vi "epx_Update Vector Color.vi"(8 "error in (no error)":errorcluster, 9 "Background Decoratin":refnum<vi>, 10 "Display State In":T1={"BGColor"=0, "FGColor"=0, "GridColor"=9868950, "Number of Polar Grids"=12, "Number of Circle Grids"=4, "Vector.Active"=0, "Vectors.Properties"=[], "Height"=0, "Width"=0} {"Number of Circle Grids" min=1 max=100 step=1; "Number of Polar Grids" min=1 max=100 step=1}, 11 "Vector Diagram":refnum<vi>) -> (0 "error out":errorcluster, 1 "Background Decoratin out":refnum<vi>, 3 "Vector Diagram out":refnum<vi>)   [LabVIEW 2011, in "NI_EP_Basic.lvlib" / "EPX Vector Diagram.xctl"]
uses:
  <vilib>/addons/Electrical Power/Basic/Controls/Vector Diagram/EPX Vector Diagram.xctl
  <vilib>/addons/Electrical Power/Basic/Controls/Vector Diagram/Abilities/epx_Vector Diagram State.ctl
  <vilib>/addons/Electrical Power/Basic/Controls/Vector Diagram/SubVIs/epx_Vector Type.ctl
  <vilib>/addons/Electrical Power/Basic/NI_EP_Basic.lvlib
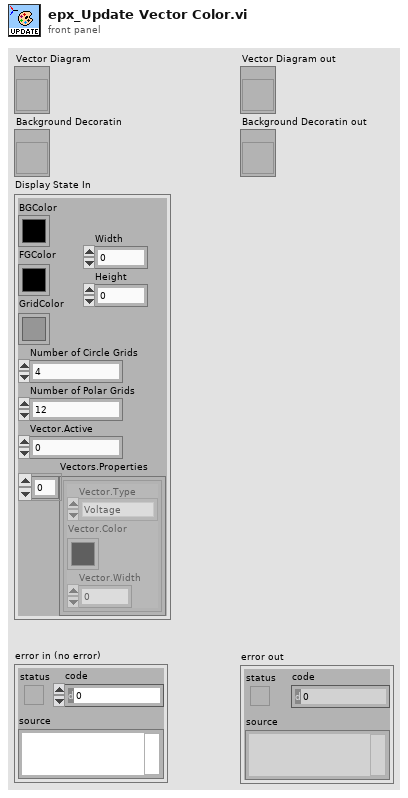
[diagram p1: front panel]
types:
  T1 = typedef "NI_EP_Basic.lvlib/EPX Vector Diagram.xctl/epx_Vector Diagram State.ctl" = cluster{"BGColor":u32, "FGColor":u32, "GridColor":u32, "Number of Polar Grids":i32, "Number of Circle Grids":i32, "Vector.Active":i32, "Vectors.Properties":cluster{"Vector.Type":T2, "Vector.Color":u32, "Vector.Width":u8}[], "Height":u32, "Width":u32}
  T2 = typedef "NI_EP_Basic.lvlib/epx_Vector Type.ctl" = enum16{"Voltage", "Current"}
  T3 = cluster{"BGColor":bool, "FGColor":bool, "GridColor":bool, "Number of Polar Grids":bool, "Number of Circle Grids":bool, "Vector.Active":bool, "Vectors.Properties":cluster{"Vector.Type":bool, "Vector.Color":bool, "Vector.Width":bool}[], "Height":bool, "Width":bool}
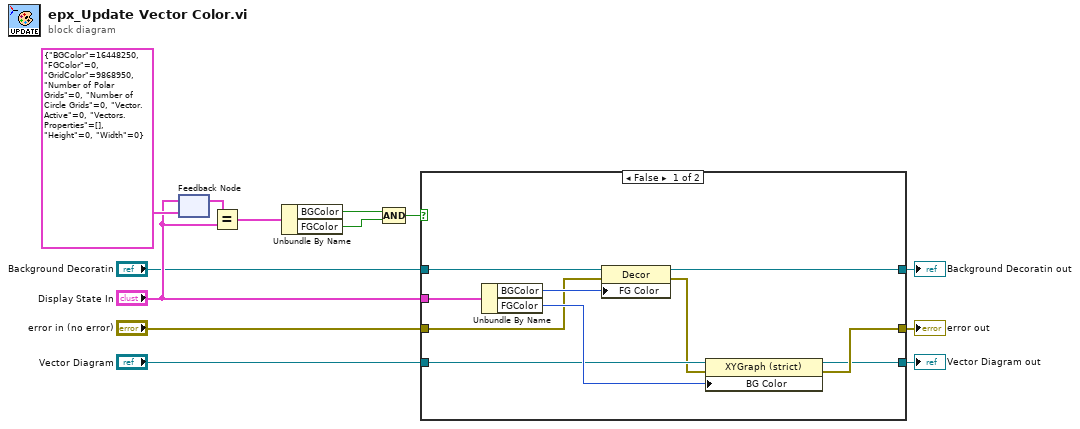
[diagram p0: block diagram]
diagram:
  n1 = feedback-in #1("Display State In") -> ()
  n2 = feedback #1(T1 {"BGColor"=16448250, "FGColor"=0, "GridColor"=9868950, "Number of Polar Grids"=0, "Number of Circle Grids"=0, "Vector.Active"=0, "Vectors.Properties"=[], "Height"=0, "Width"=0} ("Display State In")) -> (w9:T1)
  n3 = Equal?(x=w9, y="Display State In") -> (x = y?=w8:T3)
  n4 = Unbundle By Name(w8) -> ("BGColor"=w4:bool, "FGColor"=w3:bool)
  n5 = Compound Arithmetic op=AND(w4, w3) -> (w7:bool)
  n6 = case shown="False" w7 {
    tunnel: [w17 w25] -> w13
    tunnel: [w16 w26] -> w12
    tunnel: "Vector Diagram" -> [w18 w26]
    tunnel: "error in (no error)" -> [w20 w25]
    tunnel: "Display State In" -> [w21 _]
    tunnel: "Background Decoratin" -> [w19 w24]
    tunnel: [w15 w24] -> w1
    frame False {
      n7 = Unbundle By Name(w21) -> ("BGColor"=w22:u32, "FGColor"=w23:u32)
      n8 = property class="Decor"(reference=w19, error in=w20, "FG Color"=w22) -> (reference out=w15:refnum<vi>, error out=w14:errorcluster)
      n9 = property on="Property Node" class="XYGraph (strict)"(reference=w18, error in=w14, "BG Color"=w23) -> (reference out=w16:refnum<vi>, error out=w17:errorcluster)
    }
    frame True {
    }
  }
  "error out" <- w13
  "Vector Diagram out" <- w12
  "Background Decoratin out" <- w1
